vi "Test TCRS Temperature Ramping Down.vi"(8 "error in (no error)":errorcluster, 11 "Thermal Chamber Response Simlator Test In":refnum<class "Thermal Chamber Response Simlator Test.lvclass">) -> (0 "error out":errorcluster, 3 "Thermal Chamber Response Simlator Test Out":refnum<class "Thermal Chamber Response Simlator Test.lvclass">)   [LabVIEW 2020, in "Thermal Chamber Response Simlator Test.lvclass"]
uses:
  Thermal Chamber Response Simlator Test.lvclass
  C:/Program Files/National Instruments/LabVIEW 2024/vi.lib/Astemes/LUnit/Test Case.lvclass
  Thermal Chamber Response Simlator/Thermal Chamber Response Simlator.lvclass
  Thermal Chamber Response Simlator/Thermal Chamber Response Simlator.lvclass/Thermal Chamber Response Simlator.ctl
  <vilib>/Astemes/LUnit/Test Case.lvclass/Test Case.ctl
  <vilib>/Astemes/LUnit/Palette/Pass If Equal.vi/cbf50e99-f124-4847-863a-8e9794d3dede.vi
  <vilib>/Astemes/LUnit/Core/LUnit Test Case/Private/Append Pass Result.vi
  <vilib>/Astemes/LUnit/Core/LUnit Test Case/Private/Append Fail Result.vi
  <vilib>/Astemes/LUnit/Palette/Pass If Equal.vi/cbf50e99-f124-4847-863a-8e9794d3dede.vi/9c5d11cd-9439-4240-a1ee-d9baace9c924.vi
  <vilib>/Astemes/LUnit/Core/LUnit Test Case/Private/Run In UI.vi
  <vilib>/Utility/error.llb/Clear Errors.vi
  Thermal Chamber Response Simlator/Private/Get Current Time if Not Set.vi
  <vilib>/Astemes/LUnit/Test Case.lvclass
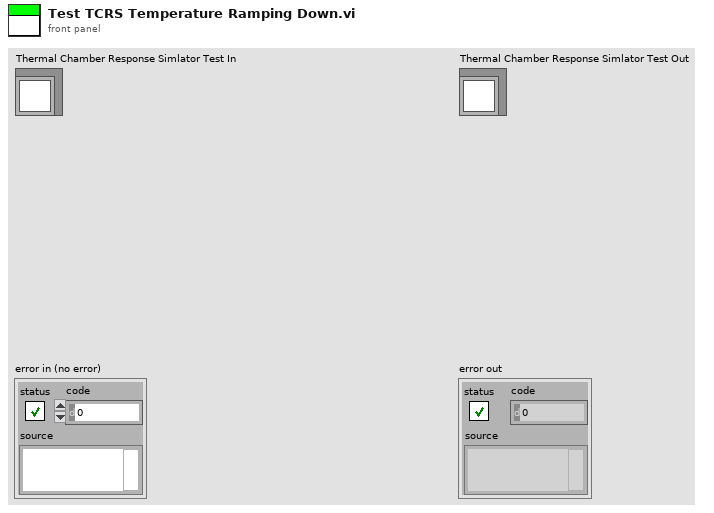
[diagram p1: front panel]
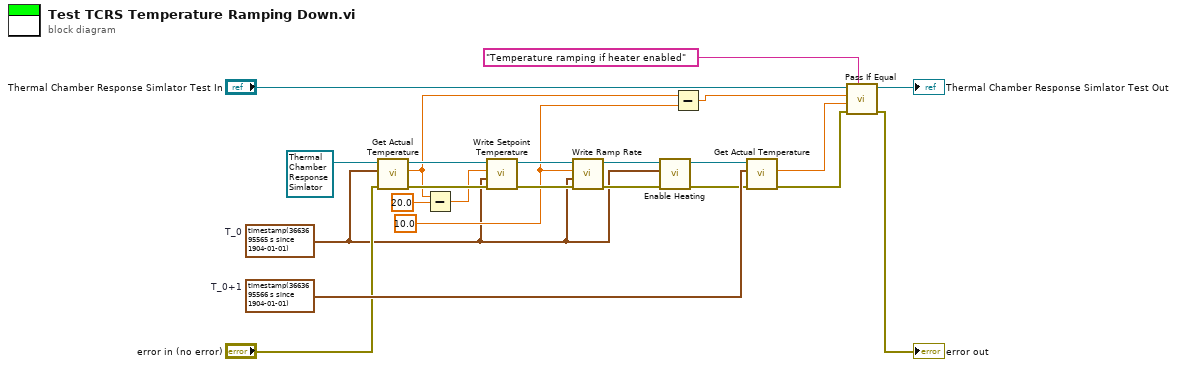
[diagram p0: block diagram]
diagram:
  w19 = timestamp(3663695566 s since 1904-01-01)  # T_0+1
  w4 = 10.0 ("Ramp Rate [degC/s]")
  w1 = timestamp(3663695565 s since 1904-01-01)  # T_0
  n1 = call "Get Actual Temperature.vi"("error in (no error)"="error in (no error)", "Time Stamp"=w1, "Thermal Chamber Response Simlator In"=refnum<class "Thermal Chamber Response Simlator.lvclass"> refnum ("Thermal Chamber Response Simlator.lvclass")) -> ("error out"=w21:errorcluster, "Actual Temperature [degC]"=w5:dbl, "Thermal Chamber Response Simlator Out"=w7:refnum<class "Thermal Chamber Response Simlator.lvclass">)  [unwired: 6 in]
  n2 = Subtract(x=w5, y=20.0) -> (x-y=w3:dbl)
  n3 = call "Write Setpoint Temperature.vi"("error in (no error)"=w21, "Update Time"=w1, "Setpoint Temperature [degC]"=w3, "Thermal Chamber Response Simlator In"=w7) -> ("error out"=w8:errorcluster, "Thermal Chamber Response Simlator Out"=w6:refnum<class "Thermal Chamber Response Simlator.lvclass">)  [unwired: 6 in]
  n4 = call "Write Ramp Rate.vi"("error in (no error)"=w8, "Time Stamp"=w1, "Ramp Rate [degC/s]"=w4, "Thermal Chamber Response Simlator In"=w6) -> ("error out"=w20:errorcluster, "Thermal Chamber Response Simlator Out"=w11:refnum<class "Thermal Chamber Response Simlator.lvclass">)  [unwired: 6 in]
  n5 = call "Enable Heating.vi"("error in (no error)"=w20, "Start Time"=w1, "Thermal Chamber Response Simlator In"=w11) -> ("error out"=w12:errorcluster, "Thermal Chamber Response Simlator Out"=w10:refnum<class "Thermal Chamber Response Simlator.lvclass">)  [unwired: 7 in]
  n6 = Subtract(x=w5, y=w4) -> (x-y=w9:dbl)
  n7 = call "Get Actual Temperature.vi"("error in (no error)"=w12, "Time Stamp"=w19, "Thermal Chamber Response Simlator In"=w10) -> ("error out"=w17:errorcluster, "Actual Temperature [degC]"=w16:dbl)  [unwired: 6 in, 1 out]
  n8 = call <vilib>:"Pass If Equal.vi"("Description"="Temperature ramping if heater enabled", "error in (no error)"=w17, "Actual"=w16, "Expected"=w9, "LUnit Test Case In"="Thermal Chamber Response Simlator Test In") -> ("error out"=→"error out":errorcluster, "LUnit Test Case Out"=→"Thermal Chamber Response Simlator Test Out":refnum<class "Thermal Chamber Response Simlator Test.lvclass">)  [unwired: 5 in]
